vi "Close_Calls.vi"() -> ()   [LabVIEW 2023]
panel:
  in  "stop":bool
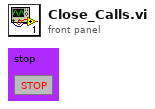
[diagram p1: front panel]
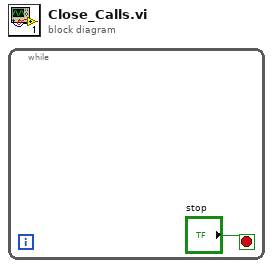
[diagram p0: block diagram]
diagram:
  n1 = while {
    stop <- "stop" stop-if-true
  }
